vi "Dispatch_Hall_Calls.vi"(8 "error in (no error)":errorcluster, 10 "Hall Calls Up/Down In":T8, 11 "Elevator Fleet in":T9) -> (0 "error out":errorcluster, 1 "Elevator Called":T1={"Door"=enum."Closed", "Person"=enum."Occupied", "Floors"={"0"=FALSE, "1"=FALSE, "2"=FALSE, "3"=FALSE}, "Up/Down/Idle"=enum."Idle", "Car Calls for Each Floor"=[FALSE, FALSE, FALSE, FALSE], "Up/Down Hall Calls for Each Floor"=[[{FALSE}, {FALSE}], [{FALSE}, {FALSE}], [{FALSE}, {FALSE}], [{FALSE}, {FALSE}], [{FALSE}, {FALSE}]], "ID"=0, "Start Timestamp"=0, "Target Duration"=0.0}, 2 "Hall Calls Up/Down Out":T8, 3 "Elevator Fleet out":T9)   [LabVIEW 2026]
uses:
  Controls/Elevator_Fleet.ctl
  Controls/Elevator_Status.ctl
  Controls/Door_Status_Enum.ctl
  Controls/Occupy_Status.ctl
  Controls/Floor_Status.ctl
  Controls/Motion_Status_Enum.ctl
  Controls/Car_Calls_Status.ctl
  Controls/Hall_Calls_Status.ctl
  Controls/Hall_Calls.ctl
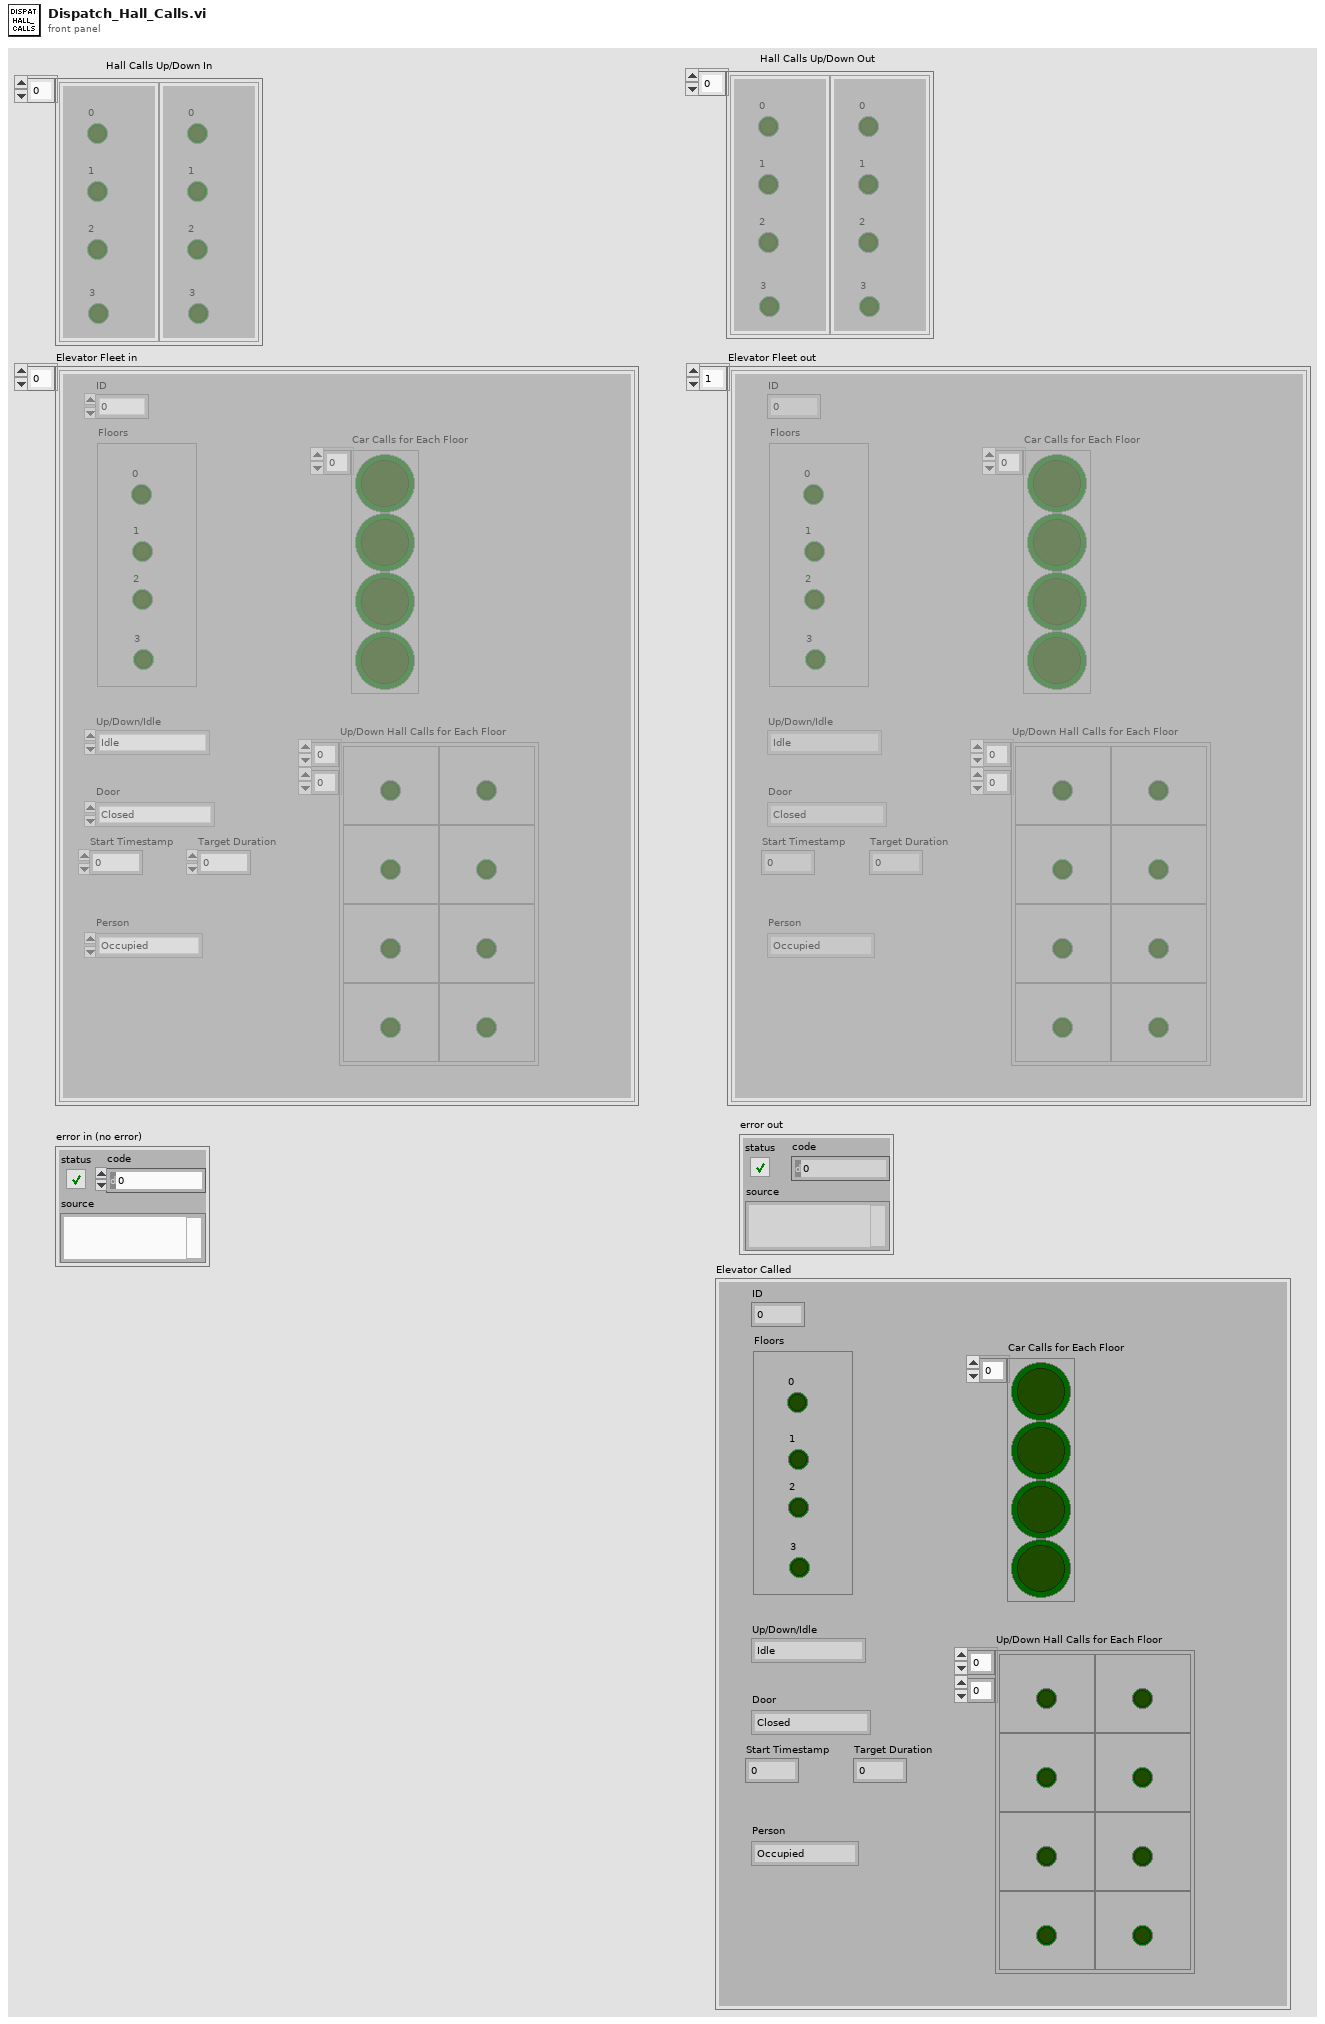
[diagram p1: front panel]
types:
  T1 = typedef "Elevator_Status.ctl" = cluster{"Door":T2, "Person":T3, "Floors":T4, "Up/Down/Idle":T5, "Car Calls for Each Floor":T6, "Up/Down Hall Calls for Each Floor":T7, "ID":i32, "Start Timestamp":u32, "Target Duration":dbl}
  T2 = typedef "Door_Status_Enum.ctl" = enum16{"Closed", "Open", "Opening", "Closing"}
  T3 = typedef "Occupy_Status.ctl" = enum16{"Occupied", "Empty"}
  T4 = typedef "Floor_Status.ctl" = cluster{"0":bool, "1":bool, "2":bool, "3":bool}
  T5 = typedef "Motion_Status_Enum.ctl" = enum16{"Idle", "Up", "Down"}
  T6 = typedef "Car_Calls_Status.ctl" = bool[]
  T7 = typedef "Hall_Calls_Status.ctl" = cluster{bool}[][]
  T8 = typedef "Hall_Calls.ctl" = cluster{"0":bool, "1":bool, "2":bool, "3":bool}[]
  T9 = typedef "Elevator_Fleet.ctl" = T1[]
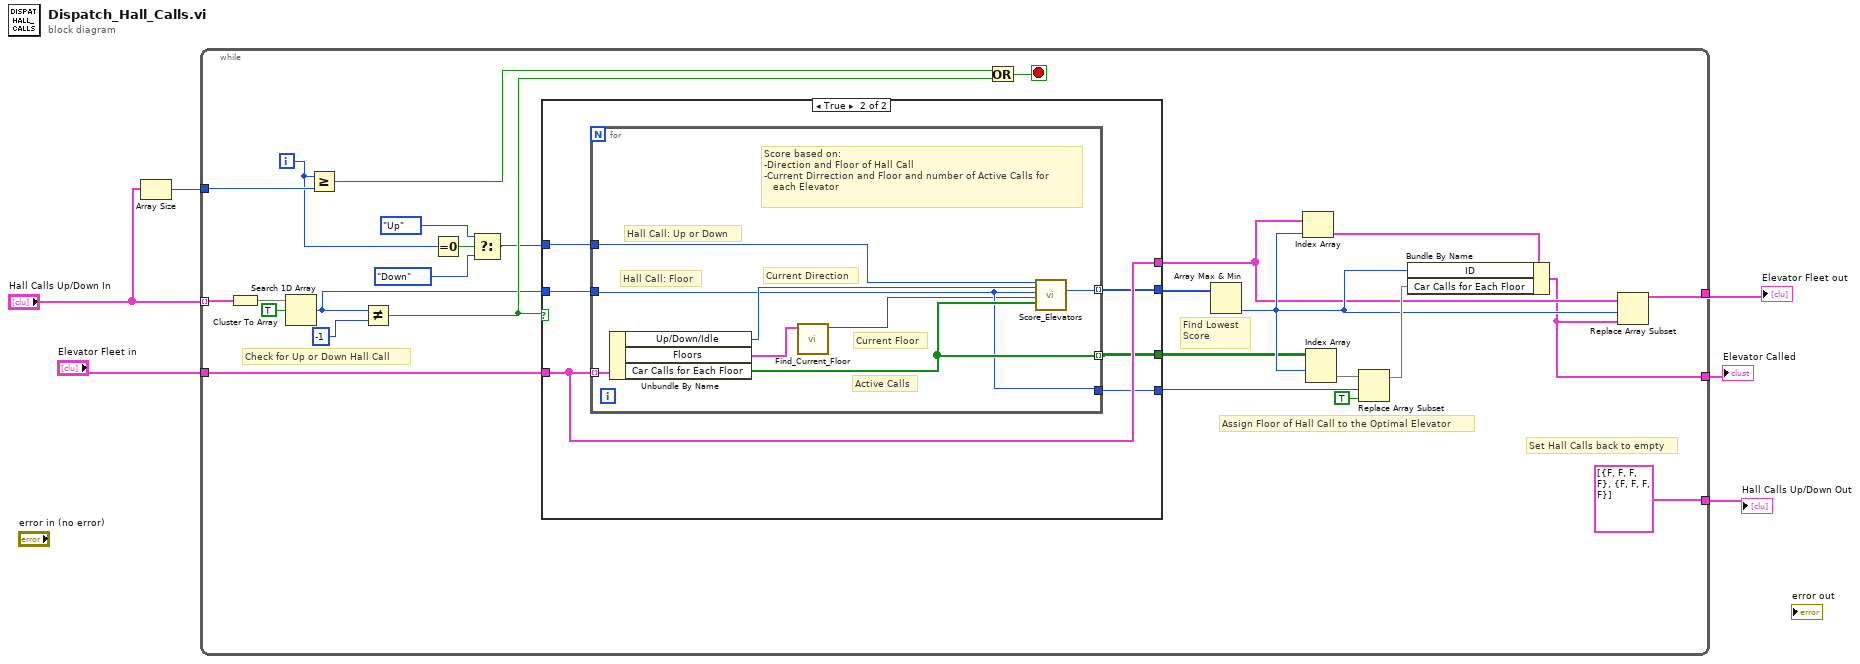
[diagram p0: block diagram]
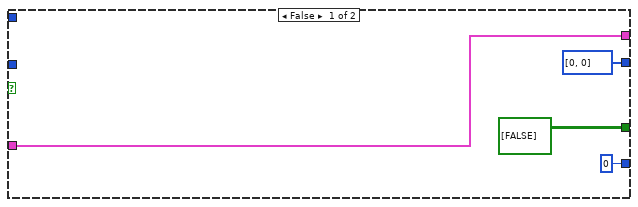
[diagram p2: hidden frame]
diagram:
  n1 = Array Size(array="Hall Calls Up/Down In") -> (size(s)=w4:i32)
  n2 = while {
    tunnel: "Elevator Fleet in" -> [w33]
    tunnel: "Hall Calls Up/Down In" -> [w19] mode=indexing
    tunnel: w4 -> [w30]
    tunnel: [w7] -> w3
    tunnel: [T8 [{"0"=FALSE, "1"=FALSE, "2"=FALSE, "3"=FALSE}, {"0"=FALSE, "1"=FALSE, "2"=FALSE, "3"=FALSE}] ("Hall Calls Up/Down Out")] -> w2
    tunnel: [w9] -> w1
    i -> [w25]
    stop <- w29 stop-if-true
    # "Find Lowest \nScore"
    # "Set Hall Calls back to empty"
    # "Assign Floor of Hall Call to the Optimal Elevator"
    # "Check for Up or Down Hall Call"
    n3 = Cluster To Array(cluster=w19) -> (array=w32:bool[])
    n4 = Search 1D Array(1D array=w32, element=TRUE) -> (index of element=w20:i32)  [unwired: 1 in]
    n5 = Greater Or Equal?(x=w25, y=w30) -> (x >= y?=w27:bool)
    n6 = Not Equal?(x=w20, y=-1) -> (x != y?=w26:bool)
    n7 = Equal To 0?(x=w25) -> (x = 0?=w22:bool)
    n8 = Select(t=Motion_Status_Enum."Up" ("Up/Down"), s=w22, f=Motion_Status_Enum."Down" ("Up/Down")) -> (s? t:f=w21:T5)
    n9 = case shown="True" w26 {
      tunnel: w33 -> [w37 w41]
      tunnel: w21 -> [_ w43]
      tunnel: w20 -> [_ w42]
      tunnel: [w37 w41] -> w13
      tunnel: [i32[] [0, 0] w40] -> w12
      tunnel: [0 ("index of element") w39] -> w11
      tunnel: [bool[][] [[FALSE]] ("Car Calls for Each Floor") w38] -> w10
      frame False {
      }
      frame True {
        n10 = for {
          tunnel: w41 -> [w51] mode=indexing
          tunnel: w43 -> [w50]
          tunnel: w42 -> [w46]
          tunnel: [w49] -> w40 mode=indexing
          tunnel: [w47] -> w38 mode=indexing
          tunnel: [w46] -> w39
          # "Score based on:\n-Direction and Floor of Hall Call\n-Current Dirrection and Floor and number of Active Calls for\n   each Elevator"
          # "Current Direction"
          # "Current Floor"
          # "Active Calls"
          # "Hall Call: Floor"
          # "Hall Call: Up or Down"
          n11 = Unbundle By Name(w51) -> ("Up/Down/Idle"=w48:T5, "Floors"=w45:T4, "Car Calls for Each Floor"=w47:T6)
          n12 = call "Find_Current_Floor.vi"("Floors"=w45) -> ("Current Floor"=w44:i32)  [unwired: 9 in, 1 out]
          n13 = call "Score_Elevators.vi"("Hall Up/Down"=w50, "Elevator Up/Down"=w48, "Desired Floor"=w46, "Current Floor"=w44, "Car Calls for Each Floor"=w47) -> ("Score"=w49:i32)  [unwired: 13 in, 1 out]
        }
      }
    }
    n14 = Or(x=w27, y=w26) -> (x .or. y?=w29:bool)
    n15 = Array Max & Min(array=w12) -> (min index (indices)=w14:i32)  [unwired: 3 out]
    n16 = Index Array(array=w13, index=w14) -> (element=w18:T1)
    n17 = Index Array(array=w10, index (row)=w14) -> (element=w17:bool[])  [unwired: 1 in]
    n18 = Replace Array Subset(array=w17, new element=TRUE ("new element/subarray"), index=w11) -> (w15:bool[])
    n19 = Bundle By Name(cluster=w18, "ID"=w14, "Car Calls for Each Floor"=w15) -> (w9:T1)
    n20 = Replace Array Subset(array=w13, new element=w9, index=w14) -> (w7:T9)
  }
  "Elevator Fleet out" <- w3
  "Hall Calls Up/Down Out" <- w2
  "Elevator Called" <- w1
